vi "选择奶茶.vi"(8 "error in (no error)":errorcluster caption="错误输入（无错误）", 9 "数值":i32=1, 10 "奶茶清单":refnum<class>[](array[class]), 11 "奶茶 输入":refnum<class "奶茶.lvclass">) -> (0 "error out":errorcluster caption="错误输出", 2 "选择的奶茶":refnum<class "奶茶.lvclass">, 3 "奶茶 输出":refnum<class "奶茶.lvclass">)   [LabVIEW 2016, in "奶茶.lvclass"]
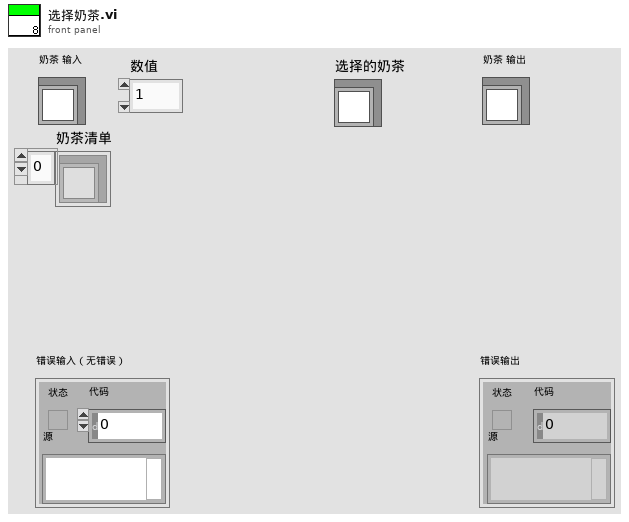
[diagram p1: front panel]
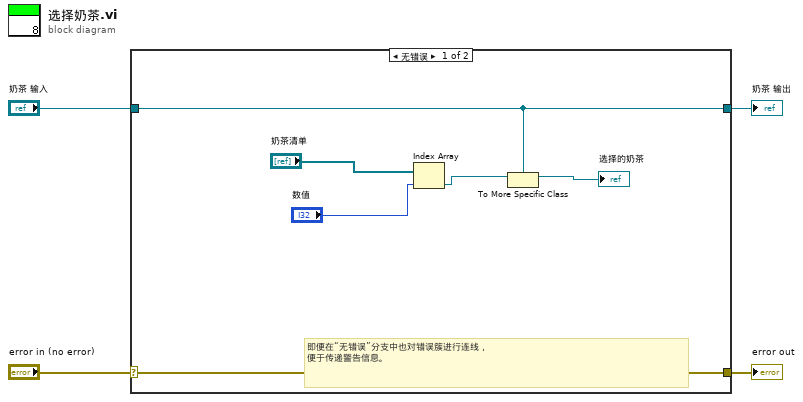
[diagram p0: block diagram]
diagram:
  n1 = case shown="无错误" "error in (no error)" {
    selector: "error in (no error)" -> [w10 w12]
    tunnel: [w10 w12] -> w3
    tunnel: [w6 w11] -> w1
    tunnel: "奶茶 输入" -> [w6 w11]
    frame No Error {
      # "即便在“无错误”分支中也对错误簇进行连线，\n便于传递警告信息。"
      n2 = Index Array(array="奶茶清单", index="数值") -> (element=w8:refnum<class>)
      n3 = To More Specific Class(target class=w6, reference=w8) -> (specific class reference=→"选择的奶茶":refnum<class "奶茶.lvclass">)  [unwired: 1 in, 1 out]
    }
    frame Error {
    }
  }
  "error out" <- w3
  "奶茶 输出" <- w1
